vi "Validate Cluster.vi"(8 "errors in":refnum<class "MultiErrors.lvclass">, 11 "Cluster":refnum<class "Cluster Config.lvclass">) -> (0 "errors out":refnum<class "MultiErrors.lvclass">)   [LabVIEW 2020, in "VolatusConfig.lvlib"]
uses:
  VolatusConfig.lvlib
  VolatusErrorUtilities/MultiErrors/MultiErrors.lvclass
  Cluster/Cluster Config.lvclass
  C:/dev/lv20CE/relink/lv-volatus/VolatusConfig/VolatusConfigElement/VolatusConfigElement.lvclass
  Meta Type.ctl
  VolatusConfigElement/VolatusConfigElement.lvclass/VolatusConfigElement.ctl
  VolatusErrorUtilities/MultiErrors/MultiErrors.lvclass/MultiErrors.ctl
  VolatusConfigElement/Element.vi
  Node/Node Config.lvclass
  lv-cdm/CDM-Config/Config Lookup/Match Meta.vi
  lv-cdm/CDM-Config/Config Element/Owner.vi
  lv-cdm/CDM-Config/Config Manager/Lookup Descendant.vi
  lv-cdm/CDM-Config/Config Filter/Config Lookup.lvclass
  VolatusConfigElement/VolatusConfigElement.lvclass
  lv-cdm/CDM-Config/Config Element/Config Element.lvclass
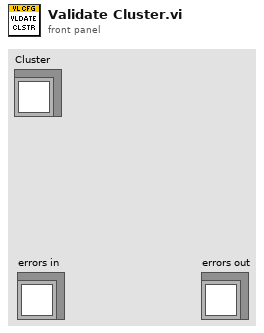
[diagram p1: front panel]
types:
  T1 = typedef "VolatusConfig.lvlib/Meta Type.ctl" = enum16{"UNKNOWN", "VL_System", "VL_Cluster", "VL_Node", "VL_Task", "VL_Group", "VL_Channel", "VL_Task_List", "VL_Scaling", "VL_Sensor", "VL_Sensor_List", "VL_Scale"}
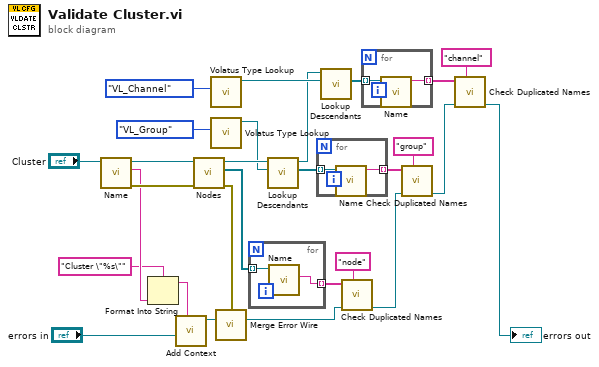
[diagram p0: block diagram]
diagram:
  n1 = call "Name.vi"("VolatusConfigElement in"="Cluster") -> ("error out"=w28:errorcluster, "Name"=w24:string, "VolatusConfigElement out"=w26:refnum<class "Cluster Config.lvclass">)  [unwired: 8 in]
  n2 = Format Into String(format string="Cluster \"%s\"", w24) -> (resulting string=w22:string)  [unwired: 2 in, 1 out]
  n3 = call "Add Context.vi"("Context"=w22, "MultiErrors in"="errors in") -> ("Added Context"=w21:refnum<class "MultiErrors.lvclass">)  [unwired: 8 in, 1 out]
  n4 = call "Nodes.vi"("error in (no error)"=w28, "Cluster in"=w26) -> ("error out"=w20:errorcluster, "Nodes"=w17:refnum<class "Node Config.lvclass">[], "Cluster out"=w15:refnum<class "Cluster Config.lvclass">)  [unwired: 7 in]
  n5 = call "Volatus Type Lookup.vi"("Meta Type"=Meta_Type."VL_Channel") -> ("Config Lookup out"=w8:refnum<class "Config Lookup.lvclass">)  [unwired: 9 in, 1 out]
  n6 = call "Volatus Type Lookup.vi"("Meta Type"=Meta_Type."VL_Group") -> ("Config Lookup out"=w13:refnum<class "Config Lookup.lvclass">)  [unwired: 9 in, 1 out]
  n7 = call "Merge Error Wire.vi"("error in (no error)"=w20, "MultiErrors in"=w21) -> ("MultiErrors out"=w16:refnum<class "MultiErrors.lvclass">)  [unwired: 13 in]
  n8 = for {
    tunnel: w17 -> [w30] mode=indexing
    tunnel: [w29] -> w19 mode=indexing
    n9 = call "Name.vi"("VolatusConfigElement in"=w30) -> ("Name"=w29:string)  [unwired: 8 in, 2 out]
  }
  n10 = call "Lookup Descendants.vi"("Lookup"=w13, "VolatusConfigElement in"=w15) -> ("Descendants"=w12:refnum<class "Config Element.lvclass">[], "VolatusConfigElement out"=w7:refnum<class "Cluster Config.lvclass">)  [unwired: 7 in, 1 out]
  n11 = for {
    tunnel: w12 -> [w32] mode=indexing
    tunnel: [w31] -> w10 mode=indexing
    n12 = call "Name.vi"("Config Element in"=w32) -> ("Name"=w31:string)  [unwired: 9 in, 1 out]
  }
  n13 = call "Lookup Descendants.vi"("Lookup"=w8, "VolatusConfigElement in"=w7) -> ("Descendants"=w4:refnum<class "Config Element.lvclass">[])  [unwired: 7 in, 2 out]
  n14 = call "Check Duplicated Names.vi"("Element Type"="node", "errors in"=w16, "Names"=w19) -> ("errors out"=w2:refnum<class "MultiErrors.lvclass">)  [unwired: 8 in]
  n15 = for {
    tunnel: w4 -> [w34] mode=indexing
    tunnel: [w33] -> w6 mode=indexing
    n16 = call "Name.vi"("Config Element in"=w34) -> ("Name"=w33:string)  [unwired: 9 in, 1 out]
  }
  n17 = call "Check Duplicated Names.vi"("Element Type"="group", "errors in"=w2, "Names"=w10) -> ("errors out"=w3:refnum<class "MultiErrors.lvclass">)  [unwired: 8 in]
  n18 = call "Check Duplicated Names.vi"("Element Type"="channel", "errors in"=w3, "Names"=w6) -> ("errors out"=→"errors out":refnum<class "MultiErrors.lvclass">)  [unwired: 8 in]
